vi "uMsg Breakdown.vi"(7 "Delimiter (>>)":string=">>", 8 "error in (no error)":errorcluster, 10 "Length (1)":i32=1, 11 "uMsg in":refnum<class "uMsg.lvclass">) -> (0 "error out":errorcluster, 1 "Remaining arguments":string, 2 "Substring":string, 3 "uMsg out":refnum<class "uMsg.lvclass">)   [LabVIEW 2023, in "uLib.lvlib" / "uMsg.lvclass"]
doc: "Split the incoming command at a certain depth."
uses:
  uMsg.lvclass
  uMsg.lvclass/uMsg.ctl
  <vilib>/Utility/error.llb/Trim Whitespace One-Sided.vi
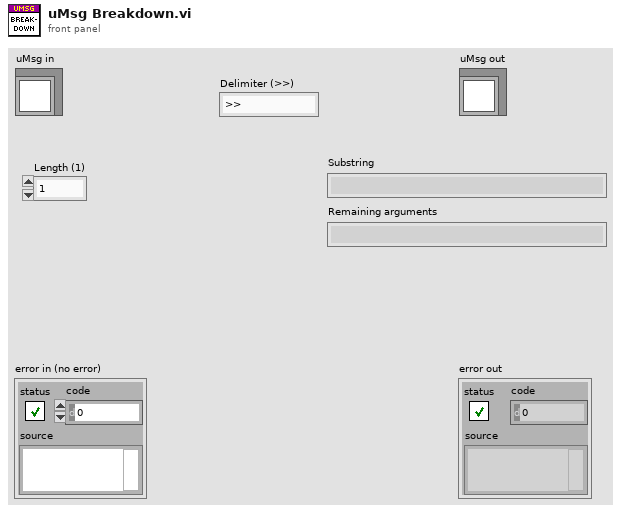
[diagram p1: front panel]
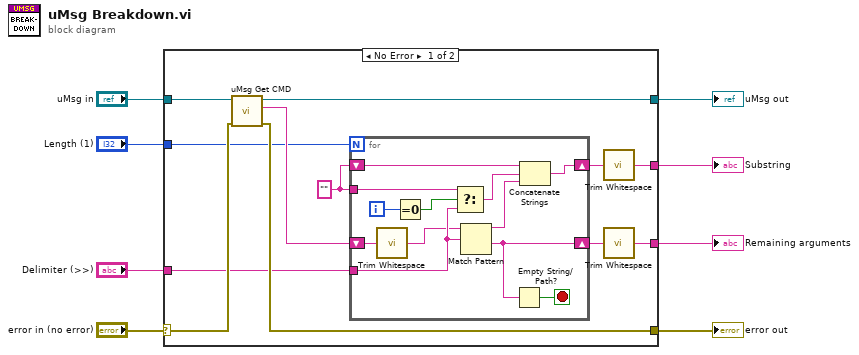
[diagram p0: block diagram]
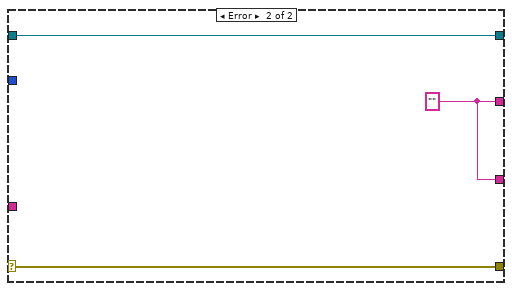
[diagram p2: hidden frame]
diagram:
  n1 = case shown="No Error" "error in (no error)" {
    selector: "error in (no error)" -> [w20 w35]
    tunnel: [w19 w35] -> w7
    tunnel: [w18 w34] -> w6
    tunnel: "uMsg in" -> [w17 w34]
    tunnel: "Delimiter (>>)" -> [w15 _]
    tunnel: [w10 w33] -> w4
    tunnel: [w9 w33] -> w3
    tunnel: "Length (1)" -> [w11 _]
    frame No Error {
      w13 = "" ("CMD")
      n2 = call "uMsg Get CMD.vi"("error in (no error)"=w20, "uMsg in"=w17) -> ("error out"=w19:errorcluster, "CMD"=w16:string, "uMsg out"=w18:refnum<class "uMsg.lvclass">)  [unwired: 7 in]
      n3 = for {
        N: w11 -> [_]
        shift-right: [w31] -> w14
        shift-left: w16 -> [w32]
        tunnel: w15 -> [w24]
        shift-right: [w30] -> w12
        shift-left: w13 -> [w26]
        tunnel: w13 -> [w25]
        i -> [w28]
        stop <- w22 stop-if-true
        n4 = call <vilib>:"Trim Whitespace.vi"("string"=w32) -> ("trimmed string"=w21:string)  [unwired: 1 in]
        n5 = Equal To 0?(x=w28) -> (x = 0?=w27:bool)
        n6 = Select(t=w25, s=w27, f=w24) -> (s? t:f=w23:string)
        n7 = Match Pattern(string=w21, regular expression=w24) -> (before substring=w29:string, after substring=w31:string)  [unwired: 1 in, 2 out]
        n8 = Empty String/Path?(string/path=w31) -> (empty?=w22:bool)
        n9 = Concatenate Strings(w26, w23, w29) -> (w30:string)
      }
      n10 = call <vilib>:"Trim Whitespace.vi"("string"=w12) -> ("trimmed string"=w10:string)  [unwired: 1 in]
      n11 = call <vilib>:"Trim Whitespace.vi"("string"=w14) -> ("trimmed string"=w9:string)  [unwired: 1 in]
    }
    frame Error {
      w33 = "" ("CMD")
    }
  }
  "error out" <- w7
  "uMsg out" <- w6
  "Remaining arguments" <- w3
  "Substring" <- w4
